vi "OffsetRect by HV and Rect Array.vi"(8 "错误输入":errorcluster, 9 "v":i16, 10 "h":i16, 11 "Rect Array":T1(array[cluster])) -> (0 "错误输出":errorcluster, 3 "OffsetRect Array":T1(array[cluster]))   [LabVIEW 2012, in "Rect Tools.lvlib"]
uses:
  Rect Tools.lvlib
  OffsetRect by HV and Rect.vi
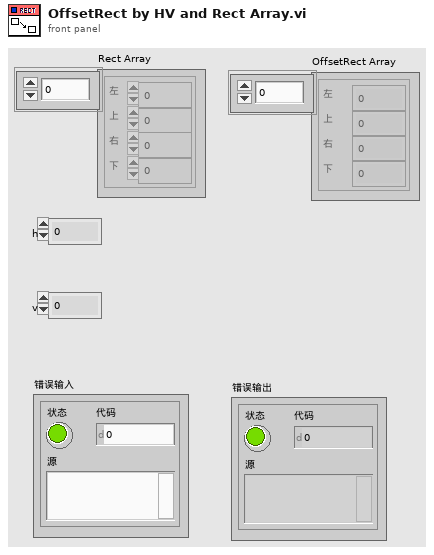
[diagram p1: front panel]
types:
  T1 = cluster{"left":i16, "top":i16, "right":i16, "bottom":i16}[]
  T2 = cluster{"left":i16, "top":i16, "right":i16, "bottom":i16}
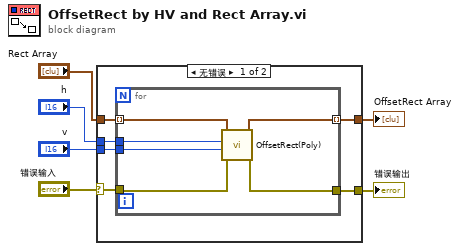
[diagram p0: block diagram]
diagram:
  n1 = case shown="无错误" "错误输入" {
    selector: "错误输入" -> [w8 w20]
    tunnel: [w7 w20] -> w5
    tunnel: "h" -> [w11 _]
    tunnel: "v" -> [w10 _]
    tunnel: "Rect Array" -> [w12 w19]
    tunnel: [w9 w19] -> w1
    frame No Error {
      n2 = for {
        tunnel: w12 -> [w16] mode=indexing
        tunnel: w11 -> [w18]
        tunnel: w10 -> [w17]
        tunnel: [w15] -> w9 mode=indexing
        tunnel: w8 -> [w14]
        tunnel: [w13] -> w7
        n3 = call-poly "OffsetRect(Poly).vi"("错误输入"=w14, "v"=w17, "h"=w18, "rect"=w16) -> ("错误输出"=w13:errorcluster, "offset rect"=w15:T2)  [unwired: 6 in]
      }
    }
    frame Error {
    }
  }
  "错误输出" <- w5
  "OffsetRect Array" <- w1
